vi "get_status_code.vi"(7 "error in (no error)":errorcluster caption="错误输入（无错误）", 10 "header":string) -> (0 "error out":errorcluster caption="错误输出", 3 "status_code":string)   [LabVIEW 2020]
panel:
  out "替换后偏移量":i32
  out "子字符串":string
  out "替换后偏移量 2":i32
  out "字符串 2":string
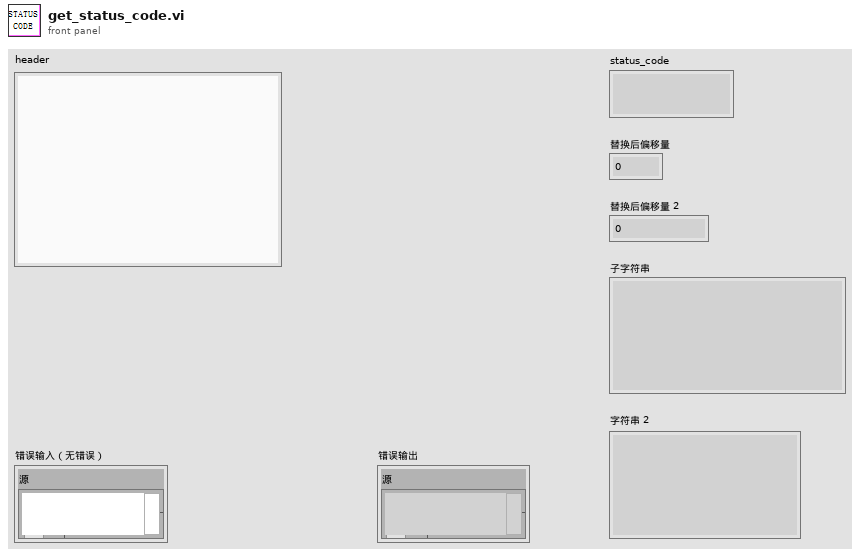
[diagram p1: front panel]
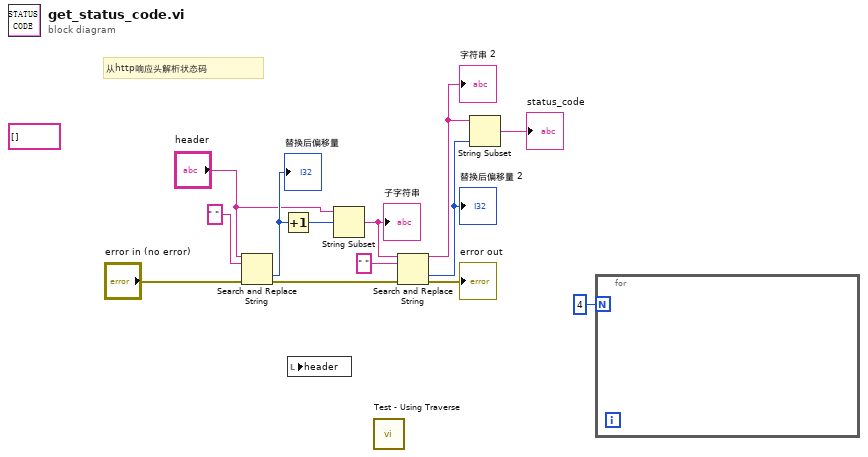
[diagram p0: block diagram]
diagram:
  (unwired) string[] []
  # "从http响应头解析状态码"
  n1 = Search and Replace String(input string="header", search string=" " ("搜索字符串"), error in="error in (no error)") -> (offset past replacement=w10:i32, error out=w3:errorcluster)  [unwired: 5 in, 2 out]
  "替换后偏移量" <- w10
  n2 = Increment(x=w10) -> (x+1=w11:i32)
  n3 = local read "header"() -> ()  [unwired: 1 in]
  n4 = String Subset(string="header", offset (0)=w11) -> (substring=w8:string)  [unwired: 1 in]
  "子字符串" <- w8
  n5 = call "Test - Using Traverse.vi"() -> ()  [unwired: 12 in]
  n6 = Search and Replace String(input string=w8, search string=" " ("搜索字符串"), error in=w3) -> (result string=w5:string, offset past replacement=w13:i32, error out=→"error out":errorcluster)  [unwired: 5 in, 1 out]
  "字符串 2" <- w5
  "替换后偏移量 2" <- w13
  n7 = String Subset(string=w5, length (rest)=w13) -> (substring=→"status_code":string)  [unwired: 1 in]
  n8 = for {
    N: 4 -> [_]
  }
